vi "Wait for Signal.vi"(4 "Error In":errorcluster, 6 "Timeout":dbl[unit]=10.0, 7 "Notifier Name":string) -> (0 "Error Out":errorcluster, 3 "Signal Data":variant)   [LabVIEW 2015, in "not_Generic Named Notifier.lvlib"]
uses:
  not_Generic Named Notifier.lvlib
  <vilib>/Utility/error.llb/Error Cluster From Error Code.vi
  <vilib>/ErrorRing/Error Ring.xnode
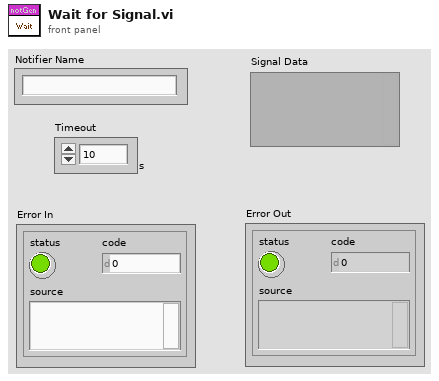
[diagram p1: front panel]
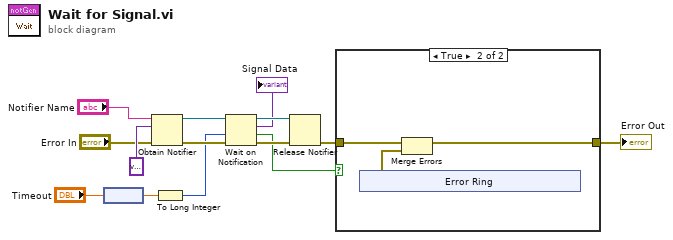
[diagram p0: block diagram]
diagram:
  n1 = node("Timeout") -> (w8:dbl)
  n2 = Obtain Notifier(name (unnamed)="Notifier Name", notification data type=variant ("element data type"), error in (no error)="Error In") -> (notifier out=w13:refnum<notifier>, error out=w14:errorcluster)  [unwired: 1 in, 1 out]
  n3 = To Long Integer(number=w8) -> (32bit integer=w7:i32)
  n4 = Wait on Notification(notifier=w13, timeout in ms (-1)=w7, error in (no error)=w14) -> (notifier out=w12:refnum<notifier>, notification=→"Signal Data":variant, timed out?=w6:bool, error out=w11:errorcluster)  [unwired: 1 in]
  n5 = Release Notifier(notifier=w12, error in (no error)=w11) -> (error out=w5:errorcluster)  [unwired: 1 in, 2 out]
  n6 = case shown="True" w6 {
    tunnel: w5 -> [w15 w18]
    tunnel: [w15 w17] -> w4
    frame False {
    }
    frame True {
      n7 = xnode "Error Ring"() -> ("error out"=w16:errorcluster)
      n8 = Merge Errors(w18, w16) -> (w17:errorcluster)
    }
  }
  "Error Out" <- w4
